vi "PKG_IMC_SetADCtrl.vi"(0 "handle":u32, 1 "paramloc":i32, 2 "paramStart":i32, 3 "id":i32, 5 "ADstart":dbl, 7 "ADend":dbl, 9 "ch":i32, 12 "axis":i32, 13 "paramEnd":i32) -> (4 "handle out":u32, 6 "function return":i32)   [LabVIEW 2011, in "IMC_Pkg4xxx.lvlib"]
doc: "PKG_IMC_SetADCtrl(IMC_HANDLE handle, double ADstart, double ADend, int ch, int paramloc, int axis, int paramStart, int paramEnd, int id);"
uses:
  IMC_Pkg4xxx.lvlib
  IMC_Pkg4xxx.dll
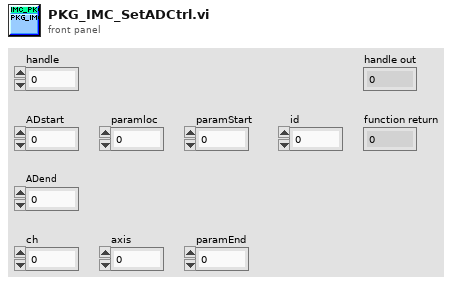
[diagram p1: front panel]
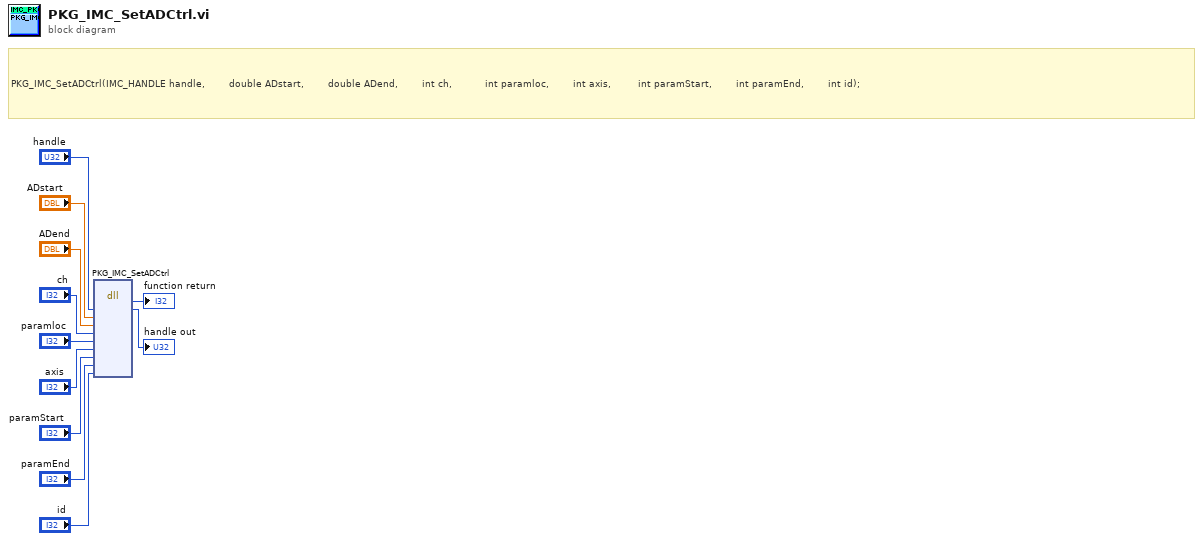
[diagram p0: block diagram]
diagram:
  # "PKG_IMC_SetADCtrl(IMC_HANDLE handle,  \t\t\t\t\t\tdouble ADstart,\t\t\t\t\t\t\t\tdouble ADend,\t\t\t\t\t\t\t\tint ch,\t\t\t\t\t\t \t\t\t\tint paramloc,\t\t\t\t\t\t\t\tint axis,\t\t\t\t\t\t\t\t\tint paramStart,\t\t\t\t\t\t\t\tint paramEnd,\t\t\t\t\t\t\t\tint id);"
  n1 = dll-call lib="PTH1mabs F光盘刻录\niMC MotionIMCNet_V4.0IMCAppincLabviewIMC_PKG4xxxIMC_PKG4xxx\nIMC_Pkg4xxx.*" fn="PKG_IMC_SetADCtrl"("handle"="handle", "ADstart"="ADstart", "ADend"="ADend", "ch"="ch", "paramloc"="paramloc", "axis"="axis", "paramStart"="paramStart", "paramEnd"="paramEnd", "id"="id") -> (→"function return":i32, "handle"=→"handle out":u32)  [unwired: 11 in, 2 out]
